vi "Parse DBL Array.vi"(6 "Seperator":string=",", 8 "error in":errorcluster, 9 "Input <JSON>":string, 10 "csv string":string, 11 "Named Columns Parser in":refnum<class "Named Fields Parser.lvclass">) -> (0 "error out":errorcluster, 2 "DBL Array":dbl[](array[numeric]), 3 "Named Columns Parser out":refnum<class "Named Fields Parser.lvclass">)   [LabVIEW 2024, in "Named Fields Parser.lvclass"]
uses:
  Named Fields Parser.lvclass
  <vilib>/JDP Science/JSONtext/LVClass Serializer/JSONtext LVClass Serializer.lvclass
  Named Fields Parser.lvclass/Named Fields Parser.ctl
  5ab44726-e38e-475a-a861-f4203e8779d1.vi
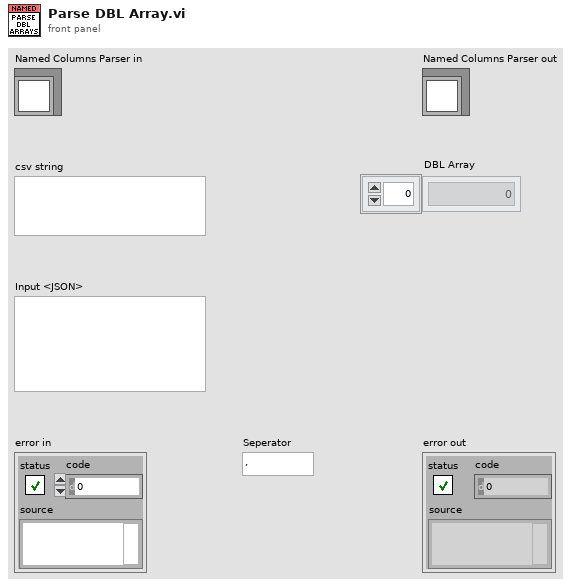
[diagram p1: front panel]
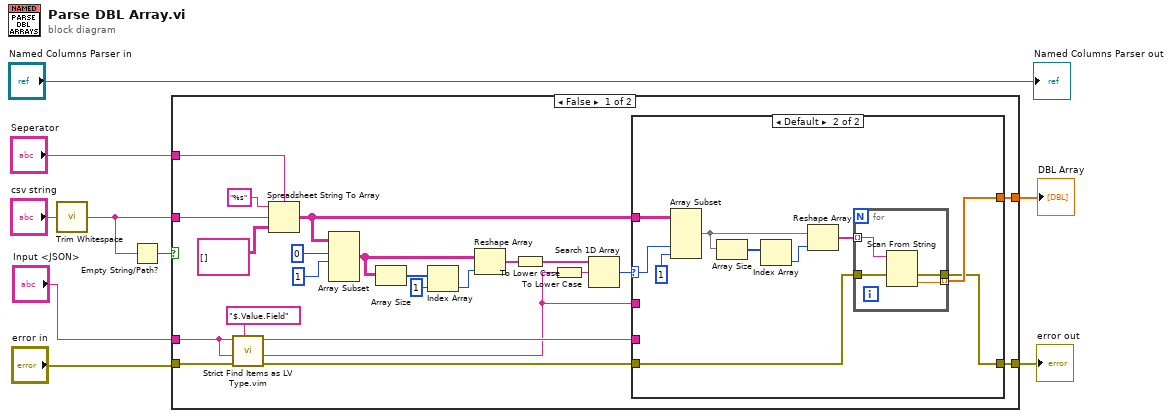
[diagram p0: block diagram]
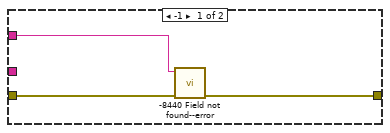
[diagram p2: hidden frame]
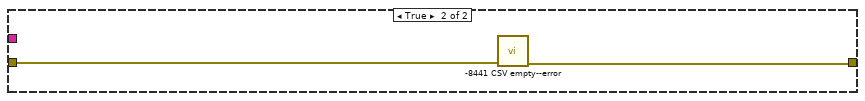
[diagram p3: hidden frame]
diagram:
  n1 = call <vilib>:"Trim Whitespace.vi"("string"="csv string") -> ("trimmed string"=w1:string)  [unwired: 1 in]
  n2 = Empty String/Path?(string/path=w1) -> (empty?=w3:bool)
  n3 = case shown="False" w3 {
    tunnel: "error in" -> [w30 w51]
    tunnel: w1 -> [w27 _]
    tunnel: [w26 _] -> w6
    tunnel: [w25 w50] -> w7
    tunnel: "Seperator" -> [w24 _]
    tunnel: "Input <JSON>" -> [w23 _]
    frame False {
      n4 = call "Strict Find Items as LV Type.vim"("$Path or Item Name"="$.Value.Field", "error in"=w30, "Data Type and Default Value"=w23, "<JSON>"=w23) -> ("error out"=w28:errorcluster, "Data out"=w13:string, "<JSON> dup"=w15:string)  [unwired: 5 in]
      n5 = Spreadsheet String To Array(delimiter (Tab)=w24, format string="%s", spreadsheet string=w27, array type (2D Dbl)=string[][] []) -> (array=w22:string[][])
      n6 = Array Subset(array=w22, index (row)=0 ("index"), length (row)=1 ("length")) -> (w17:string[][])  [unwired: 2 in]
      n7 = Array Size(array=w17) -> (size(s)=w20:i32[])
      n8 = Index Array(array=w20, index=1) -> (element=w18:i32)
      n9 = Reshape Array(w17, w18) -> (w16:string[])
      n10 = To Lower Case(string=w16) -> (all lower case string=w11:string[])
      n11 = To Lower Case(string=w13) -> (all lower case string=w10:string)
      n12 = Search 1D Array(1D array=w11, element=w10) -> (index of element=w14:i32)  [unwired: 1 in]
      n13 = case shown="Default" w14 {
        selector: w14 -> [_ w37]
        tunnel: w28 -> [w35 w41]
        tunnel: [_ w40] -> w26
        tunnel: [w34 w39] -> w25
        tunnel: w22 -> [_ w38]
        tunnel: w15 -> [_ _]
        tunnel: w13 -> [w33 _]
        frame -1 {
          n14 = call "-8440 Field not found--error.vi"("error in"=w35, "Field Name"=w33) -> ("error out"=w34:errorcluster)  [unwired: 9 in]
        }
        frame Default {
          n15 = Array Subset(array=w38, index (col)=w37, length (col)=1 ("length")) -> (w44:string[][])  [unwired: 2 in]
          n16 = Array Size(array=w44) -> (size(s)=w45:i32[])
          n17 = Index Array(array=w45) -> (element=w43:i32)  [unwired: 1 in]
          n18 = Reshape Array(w44, w43) -> (w42:string[])
          n19 = for {
            tunnel: w41 -> [w49]
            tunnel: w42 -> [w48] mode=indexing
            tunnel: [w47] -> w40 mode=indexing
            tunnel: [w46] -> w39
            n20 = Scan From String(input string=w48, error in=w49) -> (error out=w46:errorcluster, output 1=w47:dbl)  [unwired: 3 in, 2 out]
          }
        }
      }
    }
    frame True {
      n21 = call "-8441 CSV empty--error.vi"("error in"=w51) -> ("error out"=w50:errorcluster)  [unwired: 10 in]
    }
  }
  "error out" <- w7
  "DBL Array" <- w6
  "Named Columns Parser out" <- "Named Columns Parser in"
